vi "Accountmanager.vi"(8 "error in (no error)":errorcluster, 10 "Filestate":T1, 11 "Users in":T2[](array[typedef])) -> (0 "error out":errorcluster, 3 "Users out":T2[](array[typedef]))   [LabVIEW 2015]
uses:
  Controls/user.ctl
  Controls/Filestate.ctl
  <vilib>/Utility/file.llb/Read Delimited Spreadsheet (string).vi
  <vilib>/Utility/file.llb/Write Delimited Spreadsheet (string).vi
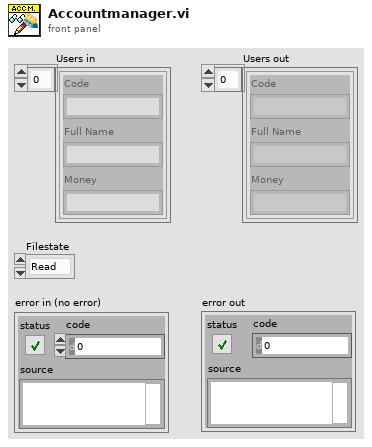
[diagram p1: front panel]
types:
  T1 = typedef "Filestate.ctl" = enum16{"Read", "Write"}
  T2 = typedef "user.ctl" = cluster{"Full Name":string, "Code":string, "Money":string}
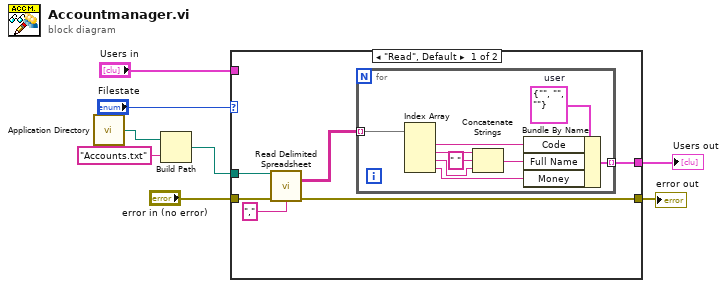
[diagram p0: block diagram]
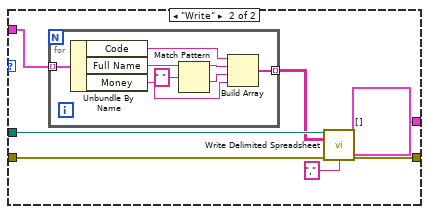
[diagram p2: hidden frame]
diagram:
  n1 = call <vilib>:"Application Directory.vi"() -> ("Application Directory"=w1:path)
  n2 = Build Path(base path=w1, name or relative path="Accounts.txt") -> (appended path=w3:path)
  n3 = case shown="\"Read\", Default" "Filestate" {
    tunnel: w3 -> [w14 w30]
    tunnel: "error in (no error)" -> [w13 w29]
    tunnel: [w10 T2[] []] -> w5
    tunnel: "Users in" -> [_ w26]
    tunnel: [w9 w28] -> w8
    frame "Read", Default {
      n4 = call-poly <vilib>:"Read Delimited Spreadsheet.vi"("file path (dialog if empty)"=w14, "error in (no error)"=w13, "delimiter (\\t)"="," ("delimiter (\\t)")) -> ("all rows"=w11:string[][], "error out"=w9:errorcluster)  [unwired: 7 in, 4 out]
      n5 = for {
        tunnel: w11 -> [w23] mode=indexing
        tunnel: [w15] -> w10 mode=indexing
        w22 = T2 {"Full Name"="", "Code"="", "Money"=""}  # user
        n6 = Index Array(array=w23) -> (element #1=w18:string, element #2=w21:string, element #3=w19:string, element #4=w16:string)  [unwired: 4 in]
        n7 = Concatenate Strings(w21, " " ("string"), w19) -> (w17:string)
        n8 = Bundle By Name(cluster=w22, "Code"=w18, "Full Name"=w17, "Money"=w16) -> (w15:T2)
      }
    }
    frame "Write" {
      n9 = for {
        tunnel: w26 -> [w38] mode=indexing
        tunnel: [w31] -> w25 mode=indexing
        n10 = Unbundle By Name(w38) -> ("Code"=w35:string, "Full Name"=w36:string, "Money"=w34:string)
        n11 = Match Pattern(string=w36, regular expression=" ") -> (before substring=w32:string, after substring=w33:string)  [unwired: 1 in, 2 out]
        n12 = Build Array(w35, w32, w33, w34) -> (w31:string[])
      }
      n13 = call-poly <vilib>:"Write Delimited Spreadsheet.vi"("file path (dialog if empty)"=w30, "2D data"=w25, "error in (no error)"=w29, "delimiter (\\t)"="," ("delimiter (\\t)")) -> ("error out"=w28:errorcluster)  [unwired: 10 in, 1 out]
    }
  }
  "Users out" <- w5
  "error out" <- w8
